vi "BGREWRITEAOF.vi"(0 "TCP session out":refnum<k5>, 11 "error in":errorcluster) -> (4 "TCP session out":refnum<k5>, 6 "Data":T1, 15 "error out":errorcluster)   [LabVIEW 2023]
uses:
  SubVIs/Controls/redis-data.ctl
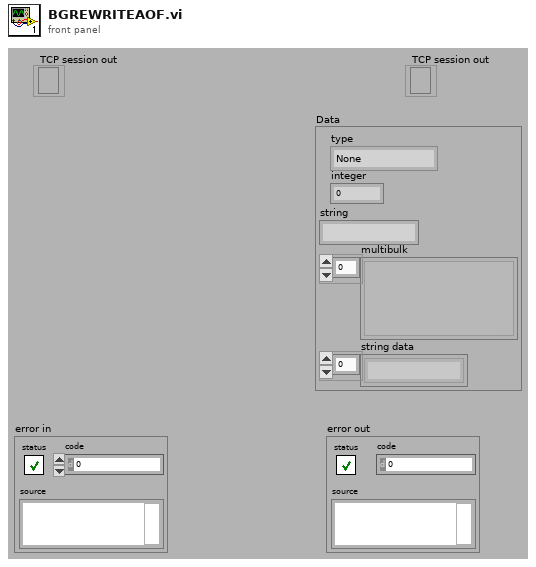
[diagram p1: front panel]
types:
  T1 = typedef "redis-data.ctl" = cluster{"type":enum16{"None", "Error", "Status", "Nil", "Integer", "String", "Multibulk"}, "integer":i64, "string":string, "multibulk":variant[], "string data":string[]}
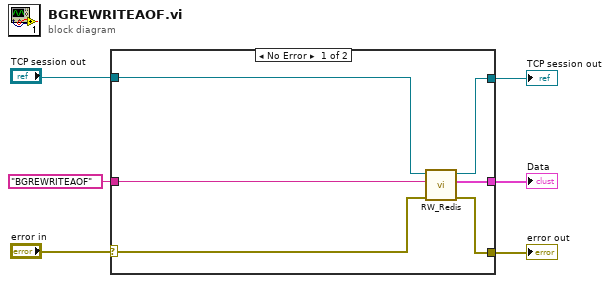
[diagram p0: block diagram]
diagram:
  n1 = case shown="No Error" "error in" {
    selector: "error in" -> [w12 w14]
    tunnel: "BGREWRITEAOF" -> [w8 _]
    tunnel: "TCP session out" -> [w9 w13]
    tunnel: [w11 w14] -> w4
    tunnel: [w10 _] -> w1
    tunnel: [w7 w13] -> w2
    frame No Error {
      n2 = call "RW_Redis.vi"("error in"=w12, "command"=w8, "TCP session in"=w9) -> ("error out"=w11:errorcluster, "Data"=w10:T1, "TCP session out"=w7:refnum<k5>)  [unwired: 6 in]
    }
    frame Error {
    }
  }
  "error out" <- w4
  "TCP session out" <- w2
  "Data" <- w1
